vi "z closure hello call.vi"(8 "error in (no error)":errorcluster, 10 "hello":cluster{}, 11 "closure":cluster{}) -> (0 "error out":errorcluster, 2 "hello out":cluster{})   [LabVIEW 2021, in "zenohc.lvlib"]
doc: "void z_closure_hello_call(const struct z_loaned_closure_hello_t *closure,\n struct z_loaned_hello_t *hello);"
uses:
  zenohc.lvlib
  zenohc.dll
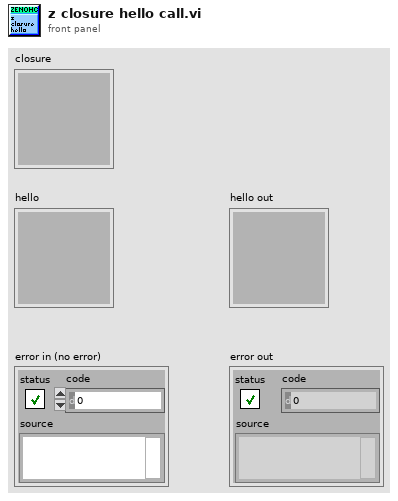
[diagram p1: front panel]
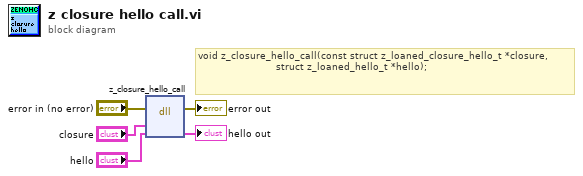
[diagram p0: block diagram]
diagram:
  # "void z_closure_hello_call(const struct z_loaned_closure_hello_t *closure,\n                          struct z_loaned_hello_t *hello);"
  n1 = dll-call lib="D:/dev/zenoh_labview/zenohc/zenohc.*" fn="z_closure_hello_call"(error in="error in (no error)", "closure"="closure", "hello"="hello") -> (error out=→"error out":errorcluster, "hello"=→"hello out":cluster{})  [unwired: 4 in, 1 out]
